vi "GOOP_VI_Item_Init.vi"(11 "Object":u64) -> ()   [LabVIEW 2014]
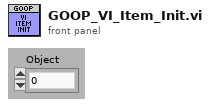
[diagram p1: front panel]
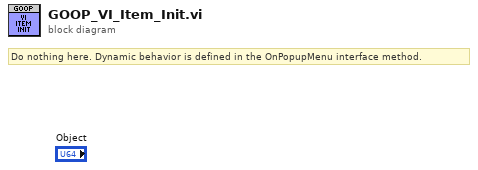
[diagram p0: block diagram]
diagram:
  # "Do nothing here. Dynamic behavior is defined in the OnPopupMenu interface method."
